vi "PPM1.vi"() -> ()   [LabVIEW 2015]
uses:
  <vilib>/Utility/miscctls.llb/LV3DPointTypeDef.ctl
  <vilib>/Simulation/Scripting/Companion Diagram/SimConfigNode/SimParams.ctl
  <vilib>/Simulation/Scripting/Companion Diagram/SimConfigNode/_simSolvers.ctl
  <vilib>/Simulation/Implementation/Shared/SIMSCR Execution Mode.ctl
  <vilib>/Simulation/Param Hierarchy/Typedefs/SIMPH Param Control Actions.ctl
  <vilib>/Simulation/Implementation/Shared/SIM limit type.ctl
  <vilib>/Simulation/Scripting/Editor Utilities/SIM subVI tag data.ctl
  <vilib>/Simulation/Scripting/Editor Utilities/SIM subVI execution type.ctl
  <vilib>/Simulation/Implementation/Shared/NILVSim_ParamChanged.vi
  <vilib>/Simulation/Implementation/Shared/NILVSIM_BeginStep.vi
  <vilib>/Simulation/Nonlinear/Implementation/NILVSim Quantizer.llb/SIM Quantizer (scalar).vi
  <vilib>/Simulation/Utility/Implementation/SIM Halt.vi
  <vilib>/Simulation/ContinuousLinear/Implementation/NILVSim Integrator new.llb/SIM Integrator distributor (scalar).vi
  <vilib>/Simulation/SignalArithmetic/Implementation/NILVSim Gain.llb/SIM Gain (vector,MatrixGain).vi
  <vilib>/Simulation/SignalDisplay/Implementation/NILVSim Time Waveform.llb/SIM Time Waveform (scalar).vi
  <vilib>/Simulation/ContinuousLinear/Implementation/NILVSim Integrator new.llb/SIM Integrator collector (scalar).vi
  <vilib>/Simulation/Implementation/Shared/SIM Fire Discrete SubVI.vi
  <vilib>/Simulation/Implementation/Shared/NILVSim_Manager.vi
  <vilib>/Utility/error.llb/Clear Errors.vi
  <vilib>/Simulation/Implementation/Shared/NILVSim_FinalizeModel.vi
  <vilib>/Simulation/Implementation/Shared/SIM Fire Discrete SubVI (Core).vi
  <vilib>/Simulation/Implementation/Shared/SIM Unbundle Sim Info.vi
  <vilib>/Simulation/Implementation/Shared/NILVSim_Initialize.vi
  <vilib>/ptbypt/Signal Generation.llb/Gaussian White Noise PtByPt.vi
  subVIs/inpparam.vi
  subVIs/matgen.vi
  subVIs/sysparam.vi
  <vilib>/Simulation/Utility/Implementation/NILVSim Get Time and IsAcceptedStep.vi
  subVIs/angset.vi
  subVIs/cdex - update quadcopter 3D model.vi
  subVIs/input.vi
  subVIs/ssa.vi
  subVIs/battery.vi
  <vilib>/Simulation/Implementation/Shared/SIMSH Read Queue.vi
  <vilib>/Simulation/Implementation/Shared/NILVSim_GetModelError.vi
  <vilib>/Simulation/Implementation/Shared/SIM Bundle Sim Info.vi
  <vilib>/Simulation/Scripting/Companion Diagram/SimConfigNode/SimDog.xnode
  <vilib>/Simulation/Implementation/XNodeFramework/SimXNode/SimX.xnode
  <vilib>/Simulation/ContinuousLinear/Implementation/NILVSim Integrator new.llb/SIM Integrator (scalar).vi
  <vilib>/ptbypt/NI_PtbyPt.lvlib
  <vilib>/Simulation/Implementation/Shared/NI_SIM_Implementation.lvlib
panel:
  out "Battery Percentage":dbl(slide) scale=0.0..100.0
  out "Current Usage":dbl
  out "Present Voltage":dbl
  out "Present Current":dbl
  out "Motors Speed":dbl[](array[slide]) scale=0.0..8000.0
  out "3D Picture Control 2":refnum<vi>(3d-picture)
  in  "Stop Button":bool
  in  "Environmental effects":dbl(slide) scale=0.0..100.0
  in  "Longitude (Y)":dbl(slide) scale=0.0..10.0
  in  "Latitude (X)":dbl(slide)
  in  "Altitude (Z)":dbl(slide)=2.0 scale=0.0..10.0
  out "X":waveform(dbl)(graph)
  out "Y":waveform(dbl)(graph)
  out "Z":waveform(dbl)(graph)
  out "Phi":waveform(dbl)(graph)
  out "Theta":waveform(dbl)(graph)
  out "Psi":waveform(dbl)(graph)
  out "Yo":dbl[](array[numeric])
  out "A":dbl[][](array[numeric])
  out "B":dbl[][](array[numeric])
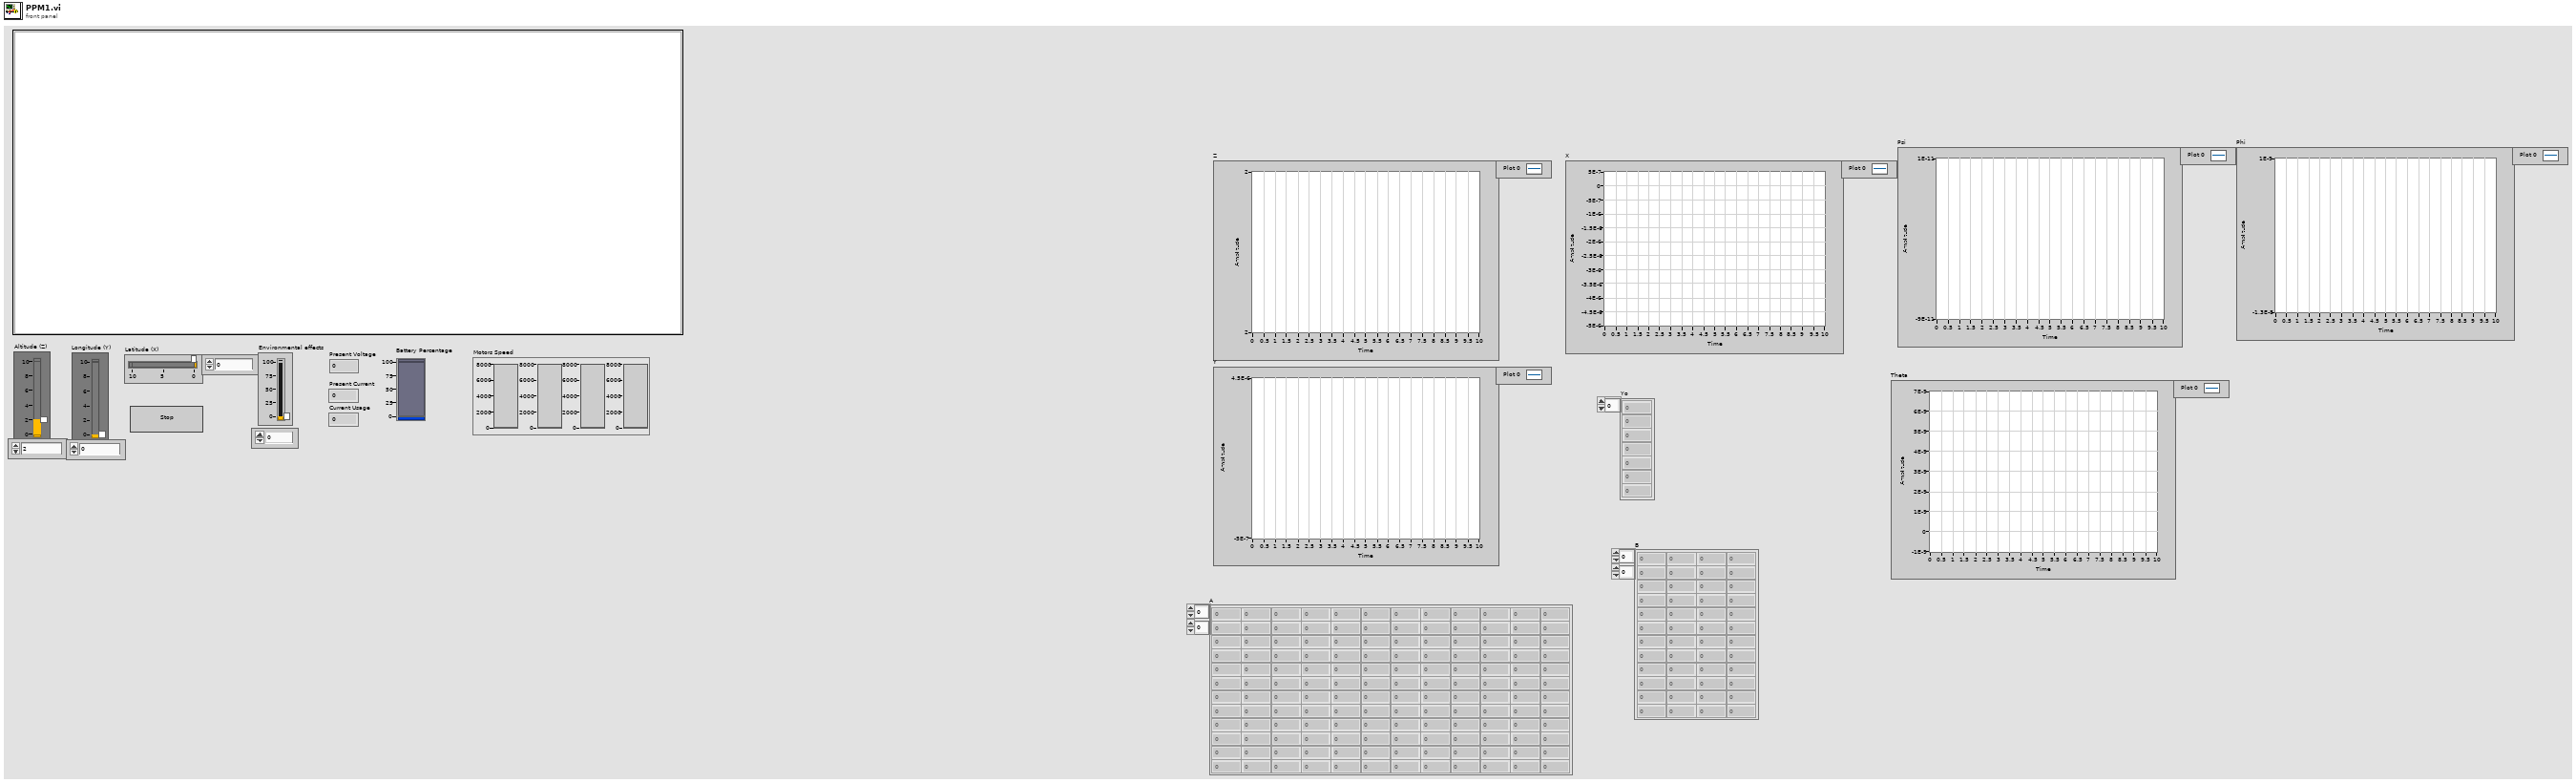
[diagram p1: front panel]
types:
  T1 = typedef "LV3DPointTypeDef.ctl" = cluster{"X":sgl, "Y":sgl, "Z":sgl}
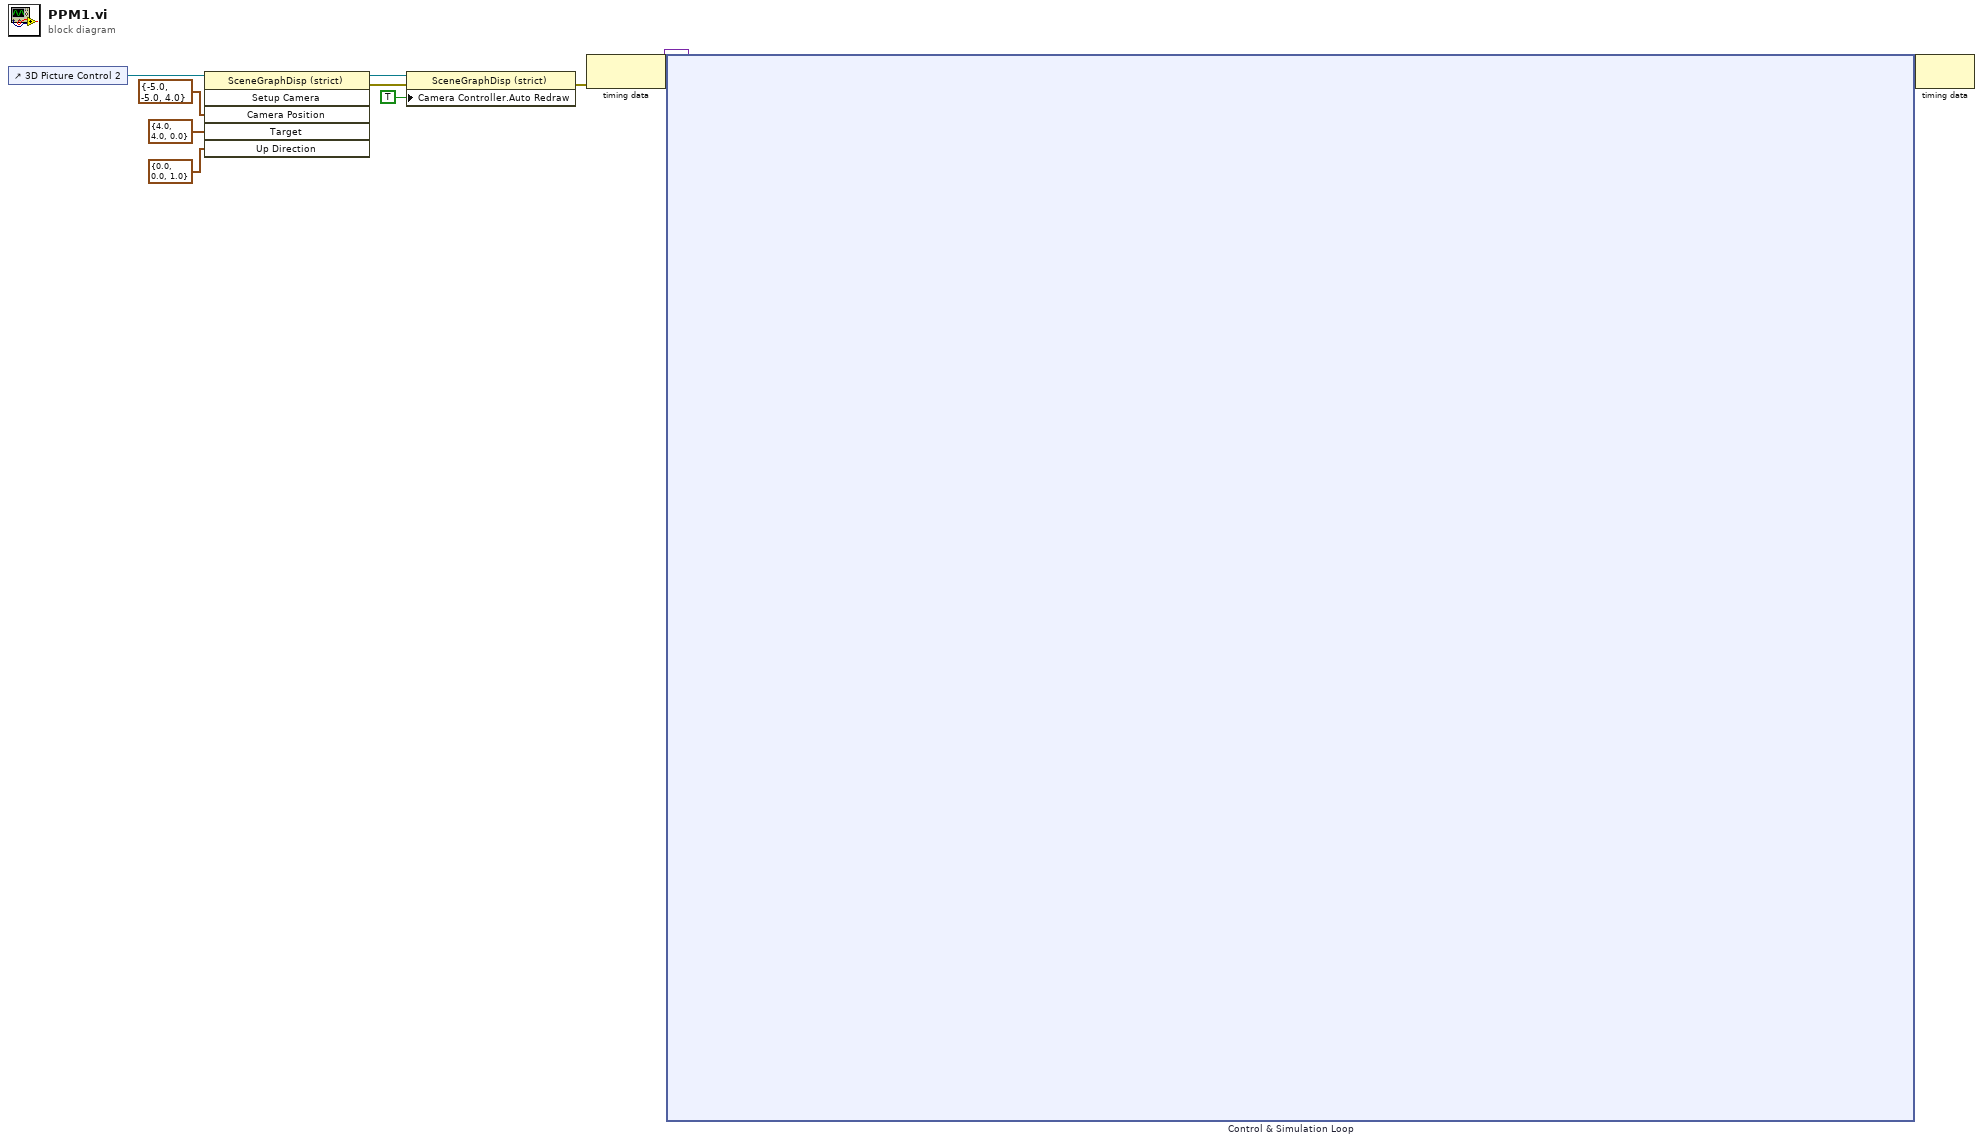
[diagram p0: block diagram]
diagram:
  n1 = control-ref of="3D Picture Control 2"() -> (w8:refnum<vi>)
  n2 = invoke on="Invoke Node" class="SceneGraphDisp (strict)" method="Setup Camera"(reference=w8, "Camera Position"=T1 {"X"=-5.0, "Y"=-5.0, "Z"=4.0}, "Target"=T1 {"X"=4.0, "Y"=4.0, "Z"=0.0}, "Up Direction"=T1 {"X"=0.0, "Y"=0.0, "Z"=1.0}) -> (reference out=w6:refnum<vi>, error out=w7:errorcluster)  [unwired: 2 in, 4 out]
  n3 = property on="Property Node" class="SceneGraphDisp (strict)"(reference=w6, error in=w7, "Camera Controller.Auto Redraw"=TRUE ("Camera Controller:Auto Redraw")) -> (error out=w1:errorcluster)  [unwired: 1 out]
  n4 = node-c288() -> (w10:variant)  [unwired: 1 in]
  n5 = node-c254 "Control & Simulation Loop"(w10, w1) -> (w9:variant)
  n6 = node-c288(w9) -> ()  [unwired: 1 out]
